vi "M-686 Reply Value.vi"(0 "VISA Pass Thru":refnum<visa-resource-name>, 7 "Cmd Reply":string, 11 "Error In":errorcluster) -> (4 "VISA Ref Dup":refnum<visa-resource-name>, 8 "Bool":bool, 10 "Value":dbl, 15 "Error Out":errorcluster)   [LabVIEW 2020]
uses:
  <vilib>/Utility/error.llb/whitespace.ctl
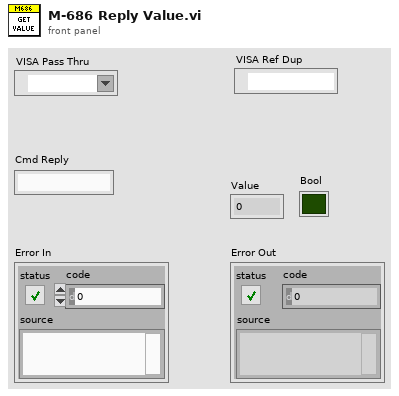
[diagram p1: front panel]
types:
  T1 = typedef "whitespace.ctl" = u16
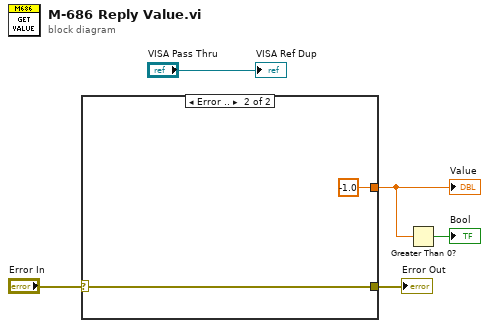
[diagram p0: block diagram]
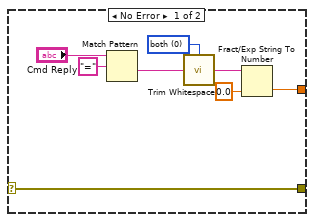
[diagram p2: hidden frame]
diagram:
  n1 = case shown="Error .." "Error In" {
    selector: "Error In" -> [w7 w15]
    tunnel: [w7 w15] -> w4
    tunnel: [w6 -1.0] -> w3
    frame No Error {
      w10 = T1 0 items=["both", "start of string", "end of string"] ("location (both)")
      n2 = Match Pattern(string="Cmd Reply", regular expression="=") -> (after substring=w11:string)  [unwired: 1 in, 3 out]
      n3 = call <vilib>:"Trim Whitespace.vi"("string"=w11, "location (both)"=w10) -> ("trimmed string"=w9:string)
      n4 = Fract/Exp String To Number(string=w9, default (0 dbl)=0.0 ("default (0 DBL)")) -> (number=w6:dbl)  [unwired: 2 in, 1 out]
    }
    frame Error {
    }
  }
  "Value" <- w3
  "Error Out" <- w4
  n5 = Greater Than 0?(x=w3) -> (x > 0?=→"Bool":bool)
  "VISA Ref Dup" <- "VISA Pass Thru"
